vi "Day4_TemplateSolution.vi"() -> ()   [LabVIEW 2026]
uses:
  <vilib>/numeric/Random Number (Range) U64.vi
  <vilib>/numeric/sub_Random U32.vi
panel:
  in  "Mode":enum32{"Simulated", "Hardware"}(radio)
  in  "Stop":bool
  in  "Buttons":bool[](array[boolean])
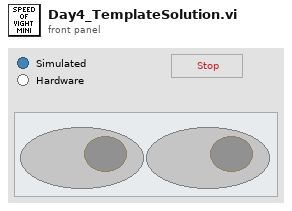
[diagram p1: front panel]
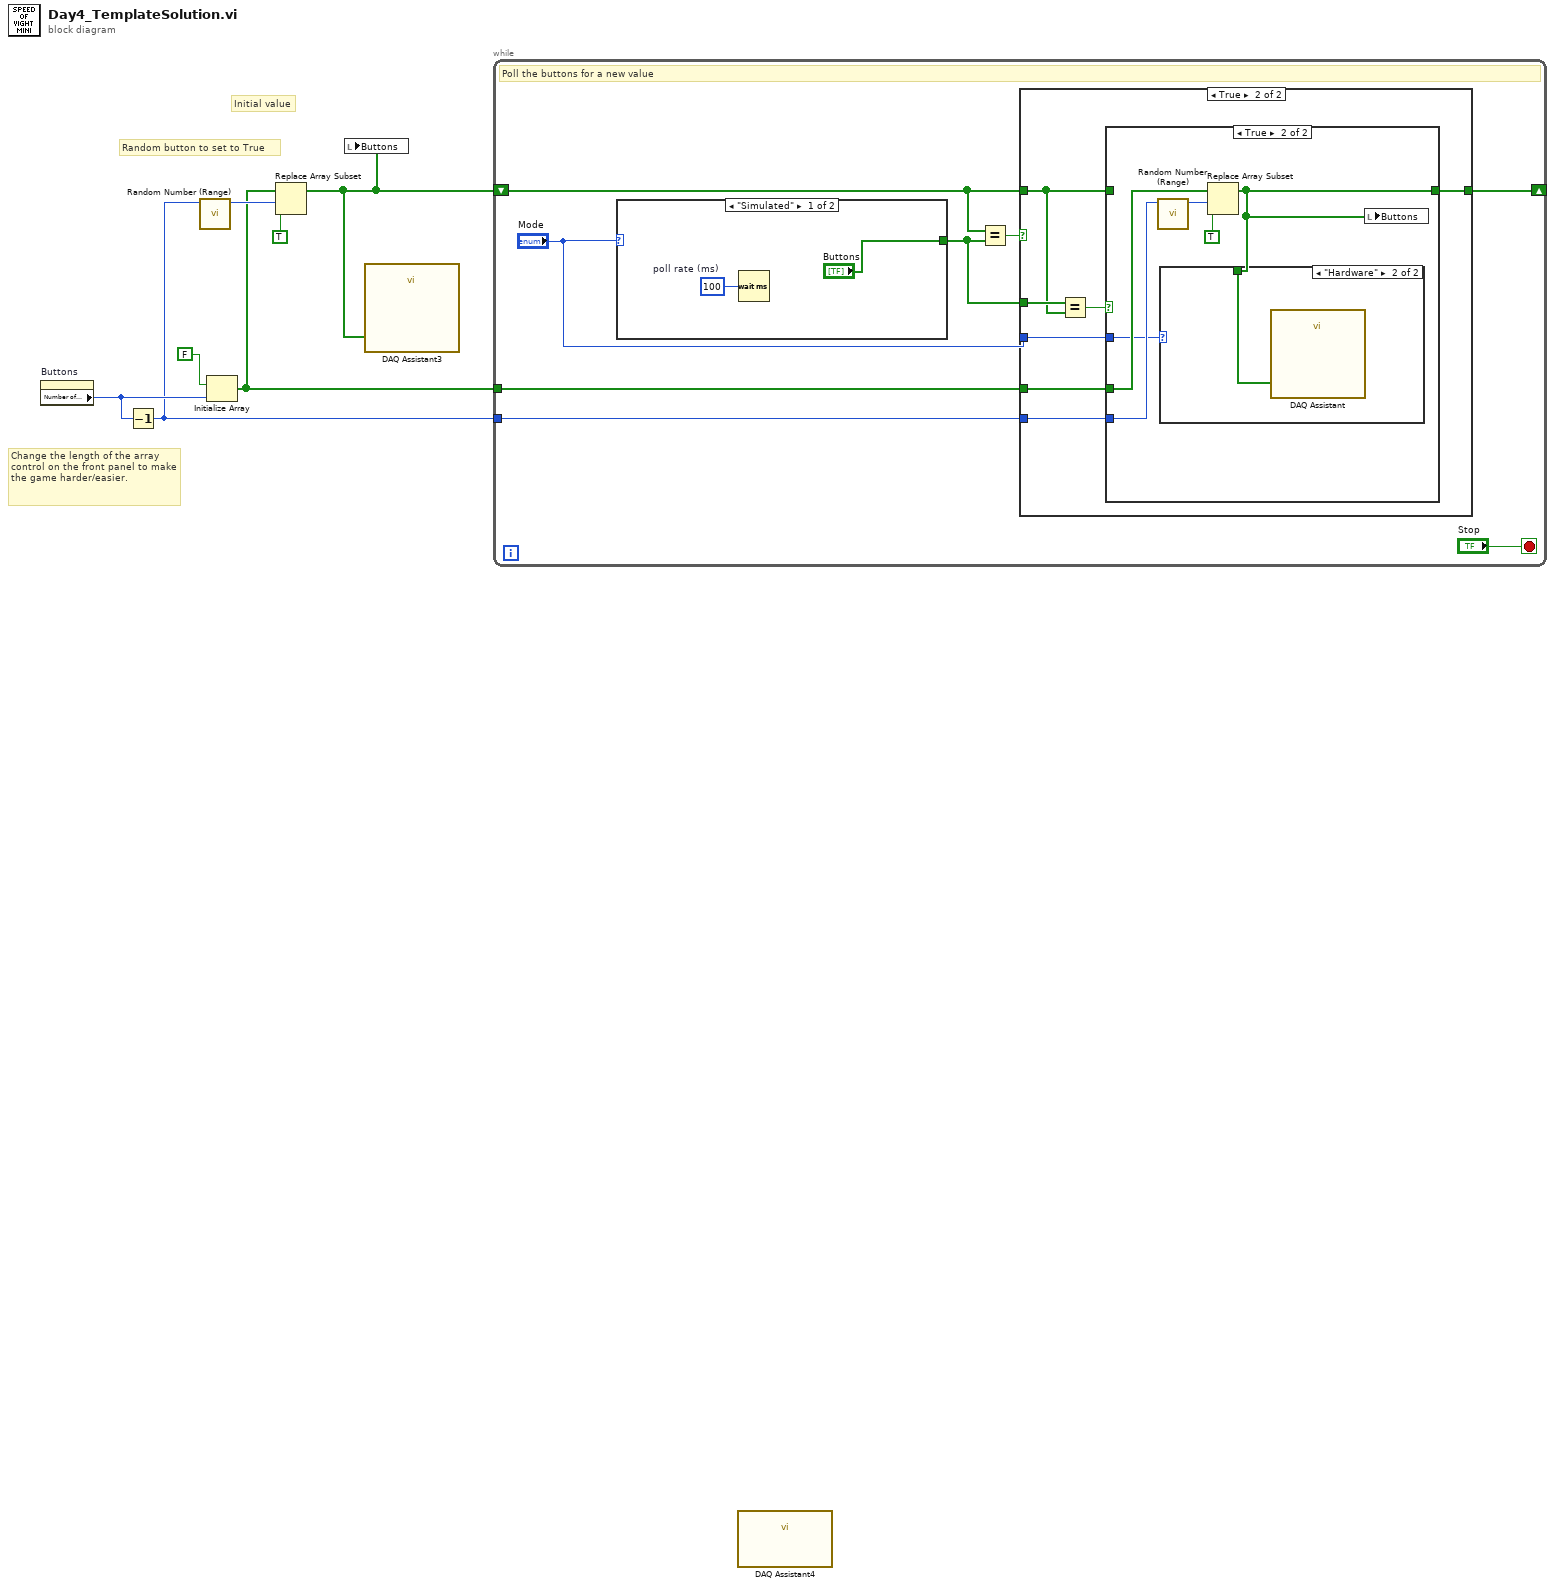
[diagram p0: block diagram]
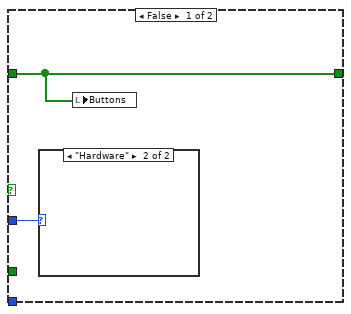
[diagram p3: hidden frame]
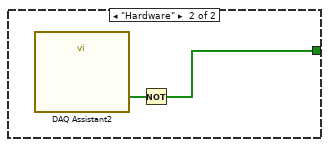
[diagram p6: hidden frame]
diagram:
  # "Random button to set to True"
  # "Initial value"
  # "Change the length of the array control on the front panel to make the game harder/easier."
  n1 = property on="Buttons" class="Arr (strict)"() -> ("Number of Columns"=w3:u32)  [unwired: 2 in, 2 out]
  n2 = Decrement(x=w3) -> (x-1=w2:u32)
  n3 = call-poly <vilib>:"Random Number (Range).vi"("upper bound (100)"=w2) -> ("number"=w6:u64)  [unwired: 10 in]
  n4 = Initialize Array(FALSE, w3) -> (w5:bool[])
  n5 = Replace Array Subset(array=w5, new element=TRUE ("new element/subarray"), index=w6) -> (w1:bool[])
  n6 = local write "Buttons"(w1) -> ()
  n7 = call "DAQ Assistant3"("data"=w1) -> ()  [unwired: 17 in, 2 out]
  n8 = while {
    tunnel: w5 -> [w11]
    shift-right: [w12] -> _
    shift-left: w1 -> [w13]
    tunnel: w2 -> [w10]
    stop <- "Stop" stop-if-true
    # "Poll the buttons for a new value"
    n9 = case shown="\"Simulated\"" "Mode" {
      tunnel: ["Buttons" w35] -> w8
      frame "Simulated" {
        w33 = u32 100  # poll rate (ms)
        n10 = Wait (ms)(milliseconds to wait=w33) -> ()  [unwired: 1 out]
      }
      frame "Hardware" {
        n11 = call "DAQ Assistant2"() -> ("data"=w36:bool[])  [unwired: 17 in, 2 out]
        n12 = Not(x=w36) -> (.not. x?=w35:bool[])
      }
    }
    n13 = Equal?(x=w13, y=w8) -> (x = y?=w14:bool)
    n14 = case shown="True" w14 {
      tunnel: w13 -> [w16 w17]
      tunnel: [w16 w20] -> w12
      tunnel: w11 -> [_ w19]
      tunnel: w8 -> [_ w23]
      tunnel: w10 -> [_ w21]
      tunnel: "Mode" -> [_ w18]
      frame False {
        # "Button value did not change"
      }
      frame True {
        # "Button value changed, see if they clicked the correct button."
        n15 = Equal?(x=w23, y=w17) -> (x = y?=w22:bool)
        n16 = case shown="True" w22 {
          tunnel: w21 -> [_ w28]
          tunnel: [w25 w26] -> w20
          tunnel: w19 -> [_ w29]
          tunnel: w17 -> [w25 _]
          tunnel: w18 -> [w24 w27]
          frame False {
            # "Wrong button clicked. Decrement score and un-click button."
            n17 = case shown="\"Hardware\"" w24 {
              frame "Simulated" {
              }
              frame "Hardware" {
              }
            }
            n18 = local write "Buttons"(w25) -> ()
          }
          frame True {
            # "Correct button clicked, update score and set a new random value"
            n19 = call-poly <vilib>:"Random Number (Range).vi"("upper bound (100)"=w28) -> ("number"=w30:u64)  [unwired: 10 in]
            n20 = Replace Array Subset(array=w29, new element=TRUE ("new element/subarray"), index=w30) -> (w26:bool[])
            n21 = case shown="\"Hardware\"" w27 {
              tunnel: w26 -> [_ w32]
              frame "Simulated" {
              }
              frame "Hardware" {
                n22 = call "DAQ Assistant"("data"=w32) -> ()  [unwired: 17 in, 2 out]
              }
            }
            n23 = local write "Buttons"(w26) -> ()
          }
        }
      }
    }
  }
  n24 = call "DAQ Assistant4"() -> ()  [unwired: 12 in]
